vi "(SubVI)Get Serial ID.vi"(8 "error in (no error)":errorcluster caption="에러 입력(에러 없음)") -> (0 "error out":errorcluster caption="에러 출력", 3 "port":string[](array[string]))   [LabVIEW 2020]
uses:
  System.Management
panel:
  out "배열 2":string[](array[string])
  out "배열":string[](array[string])
  out "Serial Port Descriptions":string[](array[string])
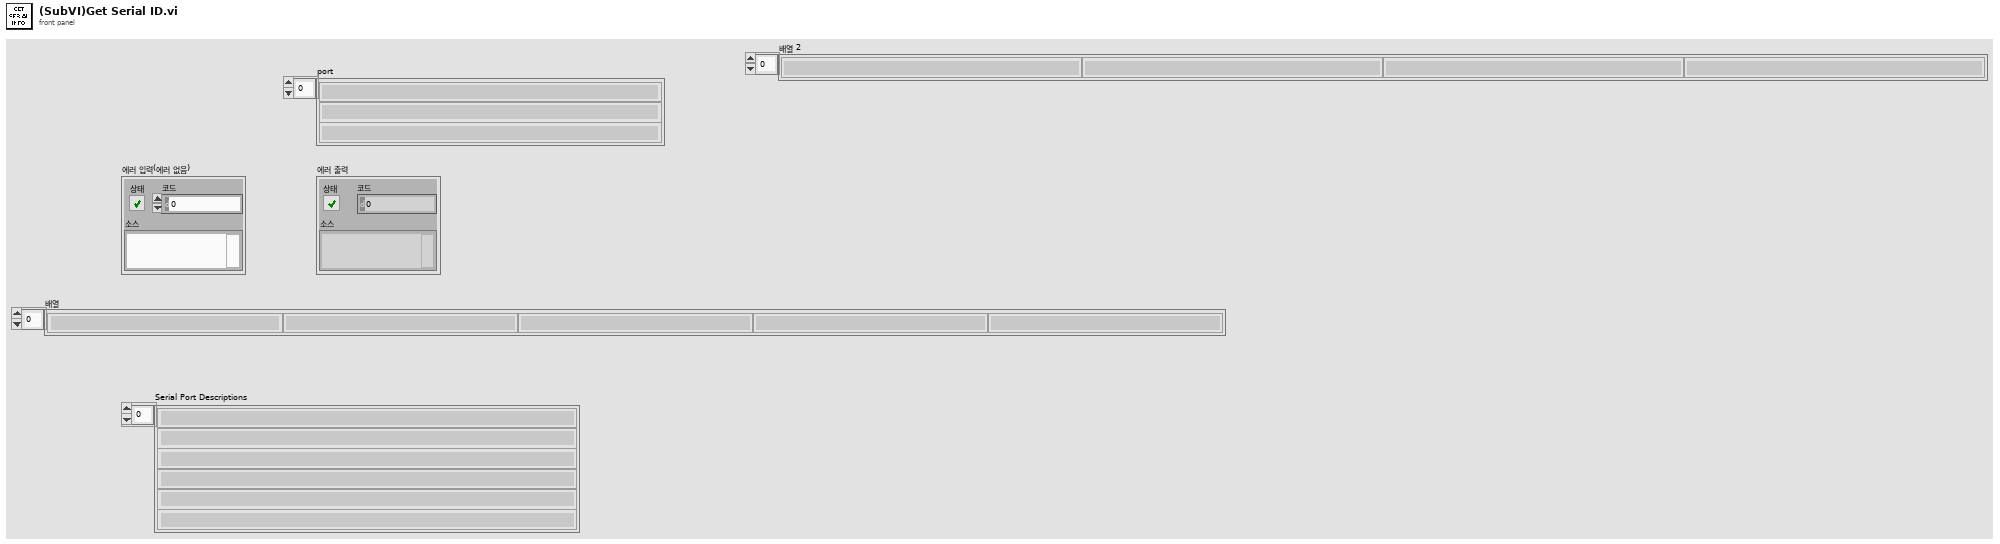
[diagram p1: front panel]
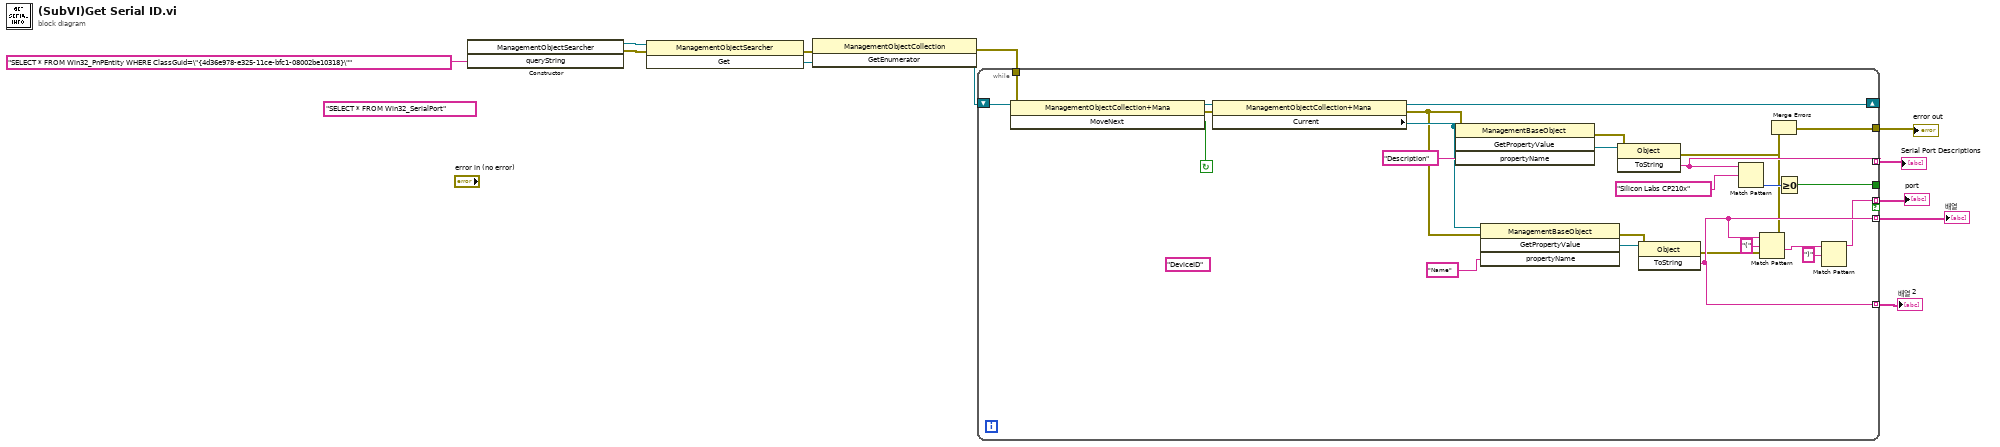
[diagram p0: block diagram]
diagram:
  (unwired) "SELECT * FROM Win32_SerialPort" ("queryString")
  n1 = constructor class="ManagementObjectSearcher"("queryString"="SELECT * FROM Win32_PnPEntity WHERE ClassGuid=\"{4d36e978-e325-11ce-bfc1-08002be10318}\"") -> (reference out=w11:refnum<k24>, error out=w12:errorcluster)  [unwired: 3 in, 2 out]
  n2 = invoke class="ManagementObjectSearcher" method="Get"(reference=w11, error in=w12) -> (error out=w3:errorcluster, "Get"=w10:refnum<k24>)  [unwired: 1 in, 1 out]
  n3 = invoke class="ManagementObjectCollection" method="GetEnumerator"(reference=w10, error in=w3) -> (error out=w2:errorcluster, "GetEnumerator"=w5:refnum<k24>)  [unwired: 1 in, 1 out]
  n4 = while {
    shift-right: [w37] -> _
    shift-left: w5 -> [w30]
    tunnel: [w34] -> w8 mode=indexing
    tunnel: [w25] -> w7 mode=indexing
    tunnel: [w31] -> _
    tunnel: [w21] -> w6 mode=indexing if=w31
    tunnel: [w25] -> w4 mode=indexing
    tunnel: w2 -> [w20]
    tunnel: [w13] -> w1
    stop <- w29 continue-if-true
    (unwired) "DeviceID" ("propertyName")
    n5 = invoke class="ManagementObjectCollection+Mana" method="MoveNext"(reference=w30, error in=w20) -> (reference out=w38:refnum<k24>, error out=w19:errorcluster, "MoveNext"=w29:bool)  [unwired: 1 in]
    n6 = property class="ManagementObjectCollection+Mana"(reference=w38, error in=w19) -> (reference out=w37:refnum<k24>, error out=w18:errorcluster, "Current"=w28:refnum<k24>)
    n7 = invoke class="ManagementBaseObject" method="GetPropertyValue"(reference=w28, error in=w18, "propertyName"="Description") -> (error out=w16:errorcluster, "GetPropertyValue"=w36:refnum<k24>)  [unwired: 1 in, 2 out]
    n8 = invoke class="ManagementBaseObject" method="GetPropertyValue"(reference=w28, error in=w18, "propertyName"="Name") -> (error out=w17:errorcluster, "GetPropertyValue"=w27:refnum<k24>)  [unwired: 1 in, 2 out]
    n9 = invoke class="Object" method="ToString"(reference=w36, error in=w16) -> (error out=w15:errorcluster, "ToString"=w34:string)  [unwired: 1 in, 1 out]
    n10 = invoke class="Object" method="ToString"(reference=w27, error in=w17) -> (error out=w14:errorcluster, "ToString"=w25:string)  [unwired: 1 in, 1 out]
    n11 = Match Pattern(string=w34, regular expression="Silicon Labs CP210x" ("정규식")) -> (offset past match=w32:i32)  [unwired: 1 in, 3 out]
    n12 = Match Pattern(string=w25, regular expression="(" ("정규식")) -> (after substring=w23:string)  [unwired: 1 in, 3 out]
    n13 = Merge Errors(w15, w14) -> (w13:errorcluster)
    n14 = Greater Or Equal To 0?(x=w32) -> (x >= 0?=w31:bool)
    n15 = Match Pattern(string=w23, regular expression=")" ("정규식")) -> (before substring=w21:string)  [unwired: 1 in, 3 out]
  }
  "Serial Port Descriptions" <- w8
  "배열" <- w7
  "port" <- w6
  "error out" <- w1
  "배열 2" <- w4
